vi "Get Control Indicator from containers.vi"(8 "error in":errorcluster, 11 "Control ref":refnum<vi>) -> (0 "error out":errorcluster, 3 "Controls[]":refnum<vi>[](array[refnum]))   [LabVIEW 2020, in "Measurement Client Wrapper.lvclass"]
uses:
  Measurement Client Wrapper.lvclass
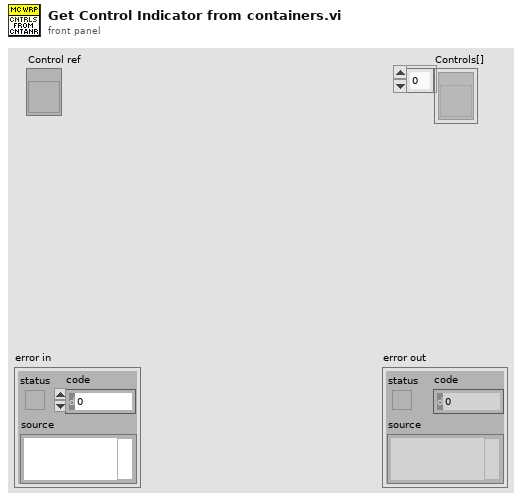
[diagram p1: front panel]
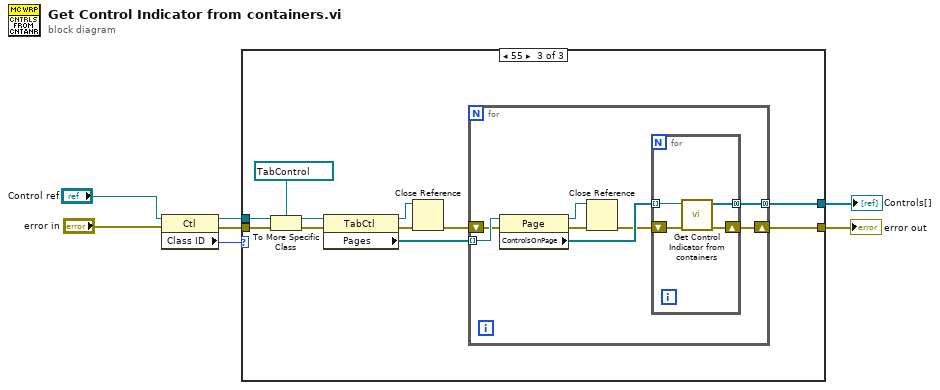
[diagram p0: block diagram]
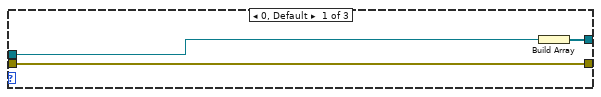
[diagram p2: hidden frame]
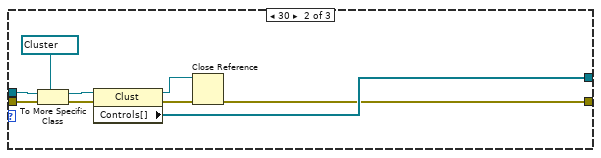
[diagram p3: hidden frame]
diagram:
  n1 = property class="Ctl"(reference="Control ref", error in="error in") -> (reference out=w3:refnum<vi>, error out=w4:errorcluster, "Class ID"=w5:u32)
  n2 = case shown="55" w5 {
    tunnel: w4 -> [w10 w17 w28]
    tunnel: [w10 w12 w23] -> w6
    tunnel: w3 -> [w9 w14 w26]
    tunnel: [w8 w13 w22] -> w7
    frame 0, Default {
      n3 = Build Array(w9) -> (w8:refnum<vi>[])
    }
    frame 30 {
      n4 = To More Specific Class(target class=refnum<vi> refnum, reference=w14, error in=w17) -> (specific class reference=w19:refnum<vi>, error out=w16:errorcluster)
      n5 = property class="Clust"(reference=w19, error in=w16) -> (reference out=w11:refnum<vi>, error out=w15:errorcluster, "Controls[]"=w13:refnum<vi>[])
      n6 = Close Reference(reference=w11, error in (no error)=w15) -> (error out=w12:errorcluster)
    }
    frame 55 {
      n7 = To More Specific Class(target class=refnum<vi> refnum, reference=w26, error in=w28) -> (specific class reference=w30:refnum<vi>, error out=w27:errorcluster)
      n8 = property class="TabCtl"(reference=w30, error in=w27) -> (reference out=w20:refnum<vi>, error out=w25:errorcluster, "Pages"=w24:refnum<vi>[])
      n9 = Close Reference(reference=w20, error in (no error)=w25) -> (error out=w21:errorcluster)
      n10 = for {
        tunnel: w24 -> [w38] mode=indexing
        shift-right: [w34] -> w23
        shift-left: w21 -> [w37]
        tunnel: [w33] -> w22 mode=concatenating
        n11 = property class="Page"(reference=w38, error in=w37) -> (reference out=w31:refnum<vi>, error out=w35:errorcluster, "ControlsOnPage"=w36:refnum<vi>[])
        n12 = Close Reference(reference=w31, error in (no error)=w35) -> (error out=w32:errorcluster)
        n13 = for {
          tunnel: w36 -> [w40] mode=indexing
          shift-right: [w41] -> w34
          shift-left: w32 -> [w42]
          tunnel: [w39] -> w33 mode=concatenating
          n14 = call "Get Control Indicator from containers.vi"("error in"=w42, "Control ref"=w40) -> ("error out"=w41:errorcluster, "Controls[]"=w39:refnum<vi>[])  [unwired: 8 in]
        }
      }
    }
  }
  "error out" <- w6
  "Controls[]" <- w7
